vi "Turret_Reset_Control.vi"(10 "Turret Is Reset":bool, 11 "Reset Turret Command":bool) -> (3 "Reset Turret Output":bool)   [LabVIEW 2012]
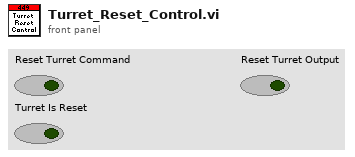
[diagram p1: front panel]
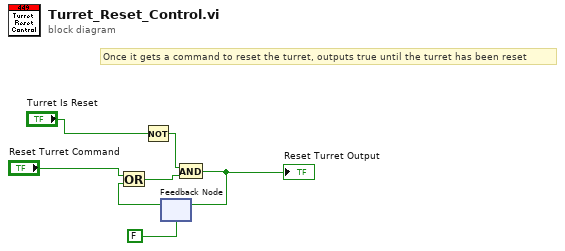
[diagram p0: block diagram]
diagram:
  # "Once it gets a command to reset the turret, outputs true until the turret has been reset"
  n1 = Not(x="Turret Is Reset") -> (.not. x?=w2:bool)
  n2 = feedback #1(FALSE ("Turret Is Reset")) -> (w6:bool)
  n3 = Or(x="Reset Turret Command", y=w6) -> (x .or. y?=w4:bool)
  n4 = And(x=w2, y=w4) -> (x .and. y?=w1:bool)
  "Reset Turret Output" <- w1
  n5 = feedback-in #1(w1) -> ()
